vi "RewriteFile(SubVI).vi"(7 "Content from file":string[](array[string]), 8 "Error In":errorcluster, 9 "Key":string, 10 "Value":string, 11 "file path (use dialog)":path) -> (0 "Error Out":errorcluster)   [LabVIEW 2018]
uses:
  <vilib>/regexp/Match Regular Expression.xnode
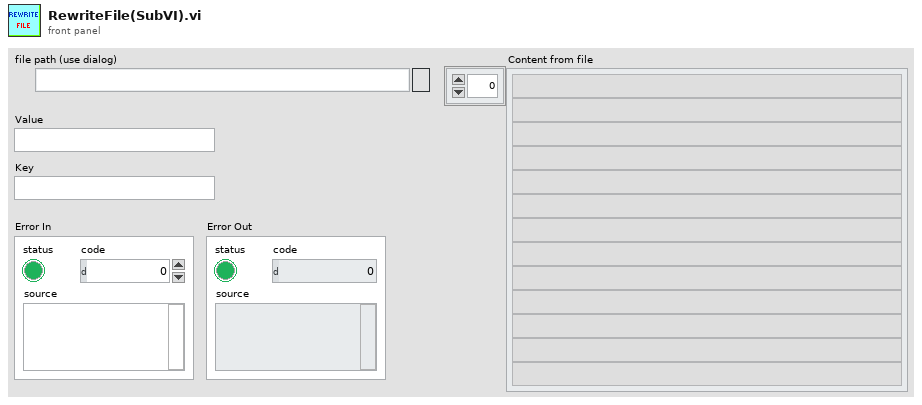
[diagram p1: front panel]
types:
  T1 = enum16{"open", "replace", "create", "open or create", "replace or create", "replace or create with confirmation"}
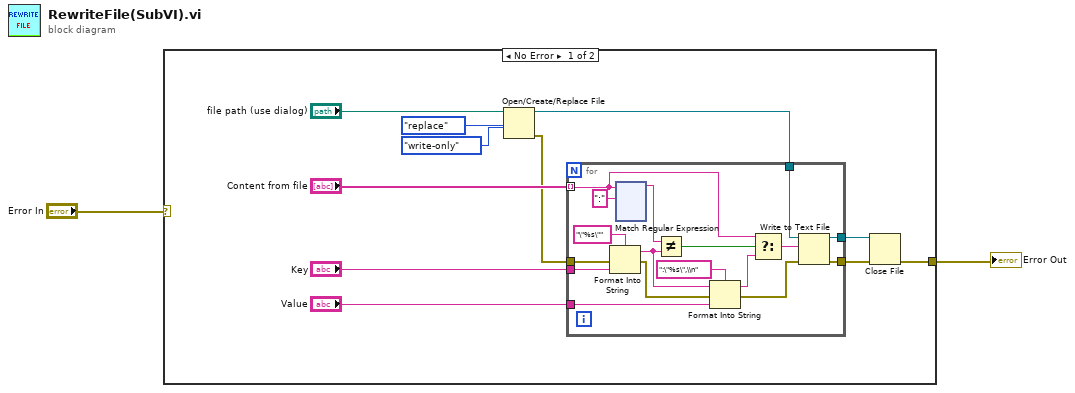
[diagram p0: block diagram]
diagram:
  n1 = case shown="No Error" "Error In" {
    selector: "Error In" -> [_ w145]
    tunnel: [w3 w145] -> w1
    frame No Error {
      n2 = Open/Create/Replace File(file path (use dialog)="file path (use dialog)", operation (0:open)=T1."replace", access (0:read/write)=enum16{"read/write", "read-only", "write-only"}."write-only") -> (refnum out=w5:refnum<file>, error out=w4:errorcluster)  [unwired: 3 in, 1 out]
      n3 = for {
        tunnel: "Content from file" -> [w22] mode=indexing
        tunnel: "Key" -> [w29]
        tunnel: "Value" -> [w24]
        tunnel: w5 -> [w21]
        tunnel: [w19] -> w8
        tunnel: [w18] -> w9
        tunnel: w4 -> [w15]
        n4 = Format Into String(format string="\"%s\"", error in=w15, w29) -> (resulting string=w25:string, error out=w17:errorcluster)  [unwired: 1 in]
        n5 = xnode "Match Regular Expression"("input string"=w22, "regular expression"=":") -> ("before match"=w14:string)  [unwired: 4 in, 4 out]
        n6 = Not Equal?(x=w14, y=w25) -> (x != y?=w27:bool)
        n7 = Format Into String(format string=":\"%s\",\\n", initial string=w25, error in=w17, w24) -> (resulting string=w23:string, error out=w16:errorcluster)
        n8 = Select(t=w22, s=w27, f=w23) -> (s? t:f=w20:string)
        n9 = Write to Text File(file (use dialog)=w21, text=w20, error in=w16) -> (refnum out=w19:refnum<file>, error out=w18:errorcluster)  [unwired: 1 in, 1 out]
      }
      n10 = Close File(refnum=w8, error in=w9) -> (error out=w3:errorcluster)  [unwired: 1 out]
    }
    frame Error {
    }
  }
  "Error Out" <- w1
